vi "test.vi"() -> ()   [LabVIEW 2023]
panel:
  out "q":i32
  out "r":i32
  out "end":i32
  in  "Size":i32
  in  "Index":i32
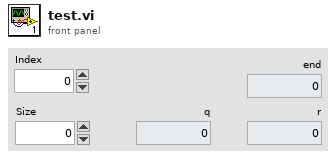
[diagram p1: front panel]
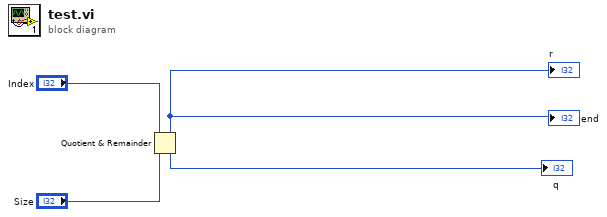
[diagram p0: block diagram]
diagram:
  n1 = Quotient & Remainder(x="Index", y="Size") -> (x-y*floor(x/y)=→"end" →"r":i32, floor(x/y)=→"q":i32)
